vi "CAN Status.vi"(7 "CAN Log Path":path, 8 "error in (no error)":errorcluster) -> (0 "error out":errorcluster, 3 "Pass?":bool)   [LabVIEW 2024]
uses:
  KvCAN/Ctrl/CAN_Operate.ctl
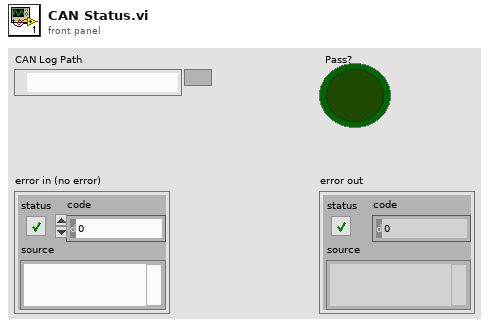
[diagram p1: front panel]
types:
  T1 = typedef "CAN_Operate.ctl" = enum16{"Init", "Write", "ReadSpecific", "Read", "Flush", "Close"}
  T2 = typedef "CAN Frame.ctl" = cluster{"TimeStamp":timestamp, "Type":u32, "Identifier":i32, "Payload":u8[]}
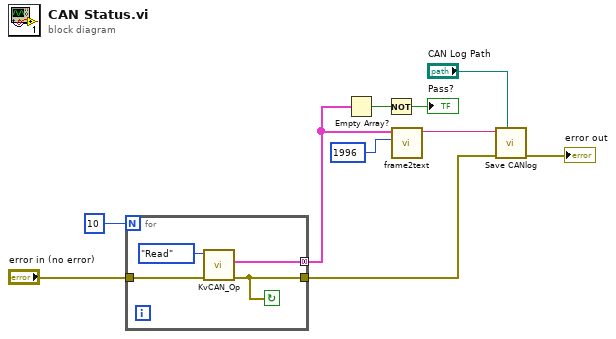
[diagram p0: block diagram]
diagram:
  n1 = for {
    N: 10 -> [_]
    tunnel: "error in (no error)" -> [w13]
    tunnel: [w11] -> w5
    tunnel: [w12] -> w6 mode=concatenating
    stop <- w11 continue-if-true
    n2 = call "KvCAN_Op.vi"("error in (no error)"=w13, "CAN Enum"=CAN_Operate."Read") -> ("error out"=w11:errorcluster, "CAN_Frame_Array"=w12:T2[])  [unwired: 5 in, 3 out]
  }
  n3 = Empty Array?(array=w6) -> (empty?=w2:bool)
  n4 = Not(x=w2) -> (.not. x?=→"Pass?":bool)
  n5 = call "frame2text.vi"("RxID"=1996, "CAN_Frame_Array"=w6) -> ("字符串"=w8:string)  [unwired: 9 in]
  n6 = call "Save CANlog.vi"("CAN Log Path"="CAN Log Path", "错误输入"=w5, "text"=w8) -> ("错误输出"=→"error out":errorcluster)  [unwired: 8 in]
